vi "Create Constr Cmd.vi"(8 "error in (no error)":errorcluster caption="错误输入（无错误）", 11 "Connncet State":T1) -> (0 "error out":errorcluster caption="错误输出", 3 "Constr":string)   [LabVIEW 2014]
uses:
  Ctr/Constr.ctl
  <vilib>/addons/database/Connection.llb/Conn ObjectReference.ctl
  <vilib>/addons/database/NI_Database_API.lvlib
  Ctr/Conneect State.ctl
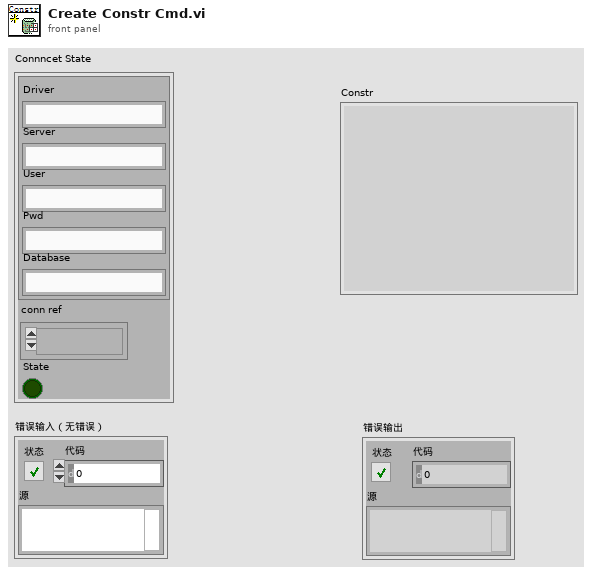
[diagram p1: front panel]
types:
  T1 = typedef "Conneect State.ctl" = cluster{"Constr":T2, "conn ref":T3, "State":bool}
  T2 = typedef "Constr.ctl" = cluster{"Driver":string, "Server":string, "User":string, "Pwd":string, "Database":string}
  T3 = typedef "NI_Database_API.lvlib/Conn ObjectReference.ctl" = refnum<k1>
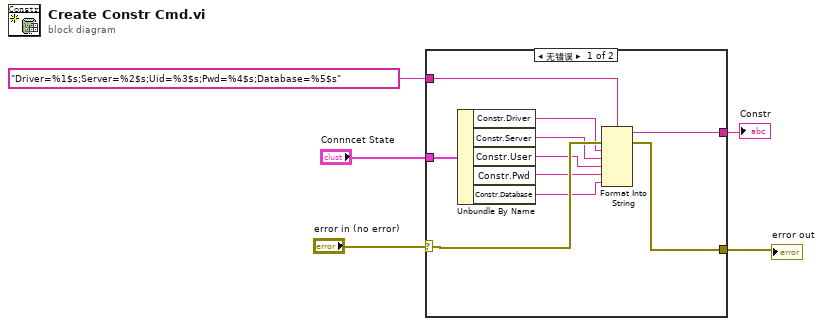
[diagram p0: block diagram]
diagram:
  n1 = case shown="无错误" "error in (no error)" {
    selector: "error in (no error)" -> [w13 w16]
    tunnel: "Connncet State" -> [w15 _]
    tunnel: "Driver=%1$s;Server=%2$s;Uid=%3$s;Pwd=%4$s;Database=%5$s" -> [w14 _]
    tunnel: [w12 w16] -> w2
    tunnel: [w6 _] -> w1
    frame No Error {
      n2 = Unbundle By Name(w15) -> ("Constr.Driver"=w11:string, "Constr.Server"=w10:string, "Constr.User"=w9:string, "Constr.Pwd"=w8:string, "Constr.Database"=w7:string)
      n3 = Format Into String(format string=w14, error in=w13, w11, w10, w9, w8, w7) -> (resulting string=w6:string, error out=w12:errorcluster)  [unwired: 1 in]
    }
    frame Error {
    }
  }
  "error out" <- w2
  "Constr" <- w1
